vi "Read ContexMenue.vi"(8 "error in (no error)":errorcluster, 11 "NotifyIcon in":refnum<class "NotifyIcon.lvclass">) -> (0 "error out":errorcluster, 2 "ContexMenue.lvclass":refnum<class "ContexMenue.lvclass">, 3 "NotifyIcon out":refnum<class "NotifyIcon.lvclass">)   [LabVIEW 2016, in "NotifyIcon.lvclass"]
uses:
  NotifyIcon.lvclass
  ContexMenue/ContexMenue.lvclass
  NotifyIcon.lvclass/NotifyIcon.ctl
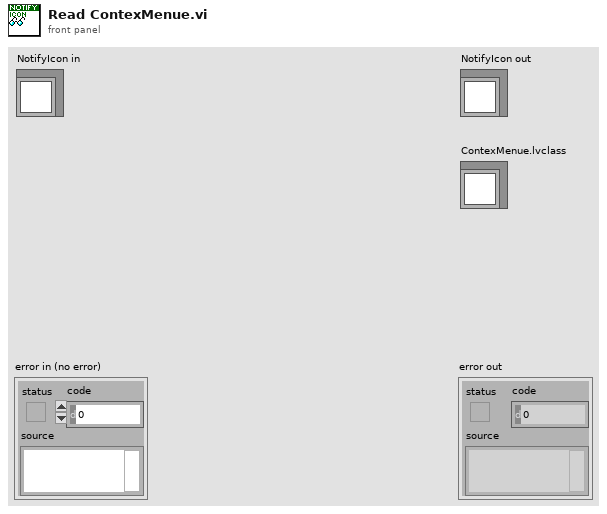
[diagram p1: front panel]
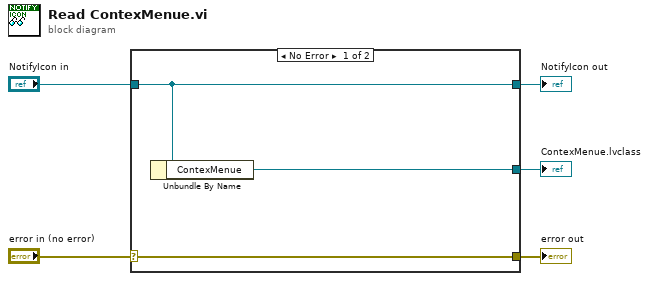
[diagram p0: block diagram]
diagram:
  n1 = case shown="No Error" "error in (no error)" {
    selector: "error in (no error)" -> [w8 w9]
    tunnel: [w8 w9] -> w4
    tunnel: [w7 w10] -> w2
    tunnel: "NotifyIcon in" -> [w7 w10]
    tunnel: [w6 _] -> w1
    frame No Error {
      n2 = Unbundle By Name(w7) -> ("ContexMenue"=w6:refnum<class "ContexMenue.lvclass">)
    }
    frame Error {
    }
  }
  "error out" <- w4
  "NotifyIcon out" <- w2
  "ContexMenue.lvclass" <- w1
